vi "Compute Max Level.vi"(0 "Moving Ripple Noise in":refnum<class "Moving Ripple Noise.lvclass">, 1 "Filter in":refnum<class "Filter.lvclass">, 5 "Level in":refnum<class "Level.lvclass">, 7 "Fs (Hz)":dbl, 9 "Vmax":dbl, 11 "error in (no error)":errorcluster) -> (4 "Moving Ripple Noise out":refnum<class "Moving Ripple Noise.lvclass">, 6 "Level thru":refnum<class "Level.lvclass">, 10 "Lmax":dbl, 15 "error out":errorcluster)   [LabVIEW 2020, in "Moving Ripple Noise.lvclass"]
uses:
  Moving Ripple Noise.lvclass
  Level/Level.lvclass
  Filter/Filter.lvclass
  Moving Ripple Noise.lvclass/Moving Ripple Noise.ctl
  e92b9aa5-16fa-470e-b09e-8802f771d522.vi
  bb50549c-138f-4f12-b68e-9a4d4622d1e5.vi
  e0497e3a-5155-4f6f-bd36-d1e8b97e81a5.vi
  1a500e8f-1266-4fc0-a246-3dcd5fe65901.vi
  Level/Read Units.vi
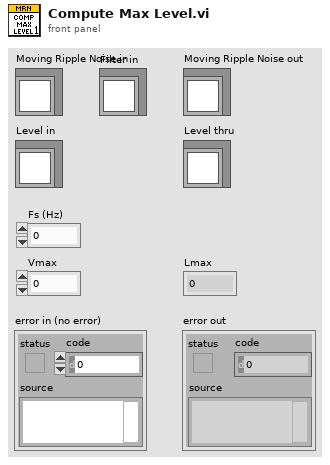
[diagram p1: front panel]
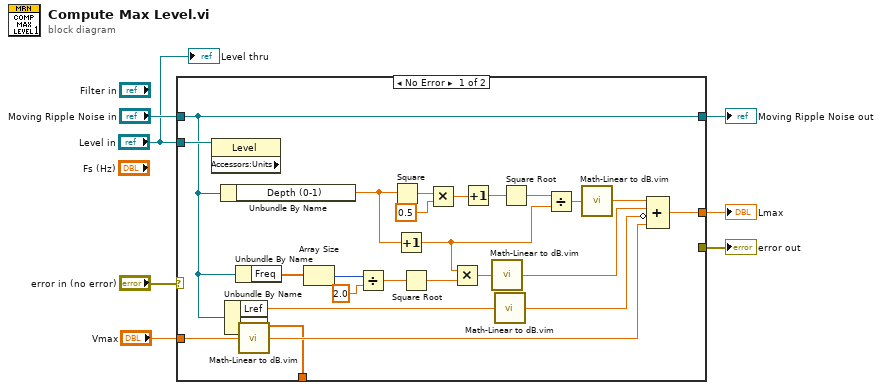
[diagram p0: block diagram]
diagram:
  n1 = case shown="No Error" "error in (no error)" {
    selector: "error in (no error)" -> [_ w32]
    tunnel: [w22 w33] -> w6
    tunnel: "Moving Ripple Noise in" -> [w22 w33]
    tunnel: "Vmax" -> [w31 _]
    tunnel: [_ w32] -> w3
    tunnel: "Level in" -> [w30 _]
    tunnel: [w11 _] -> w1
    tunnel: [w8 _] -> _
    frame No Error {
      n2 = property class="Level" props=["Accessors:Units"](reference=w30) -> ()  [unwired: 1 in, 3 out]
      n3 = Unbundle By Name(w22) -> ("Depth (0-1)"=w24:dbl)
      n4 = Unbundle By Name(w22) -> ("Lref"=w10:dbl, "A"=w8:dbl[])
      n5 = Unbundle By Name(w22) -> ("Freq"=w21:dbl[])
      n6 = call "Math-Linear to dB.vim"("linear"=w31) -> ("dB"=w12:dbl)
      n7 = Array Size(array=w21) -> (size(s)=w20:i32)
      n8 = Divide(x=w20, y=2.0) -> (x/y=w18:dbl)
      n9 = Square(x=w24) -> (x^2=w29:dbl)
      n10 = Increment(x=w24) -> (x+1=w16:dbl)
      n11 = Square Root(x=w18) -> (sqrt(x)=w17:dbl)
      n12 = Multiply(x=w29, y=0.5) -> (x*y=w28:dbl)
      n13 = Multiply(x=w16, y=w17) -> (x*y=w15:dbl)
      n14 = Increment(x=w28) -> (x+1=w27:dbl)
      n15 = call "Math-Linear to dB.vim"("linear"=w15) -> ("dB"=w13:dbl)
      n16 = call "Math-Linear to dB.vim"("linear"=w10) -> ("dB"=w9:dbl)
      n17 = Square Root(x=w27) -> (sqrt(x)=w26:dbl)
      n18 = Divide(x=w26, y=w16) -> (x/y=w23:dbl)
      n19 = call "Math-Linear to dB.vim"("linear"=w23) -> ("dB"=w14:dbl)
      n20 = Compound Arithmetic op=ADD(w14, w13, invert w9, w12) -> (w11:dbl)
    }
    frame Error {
    }
  }
  "error out" <- w3
  "Moving Ripple Noise out" <- w6
  "Lmax" <- w1
  "Level thru" <- "Level in"
